vi "createCommandList.vi"(8 "error in (no error)":errorcluster, 10 "Parameters":u32[](array[numeric]), 11 "Burst in":refnum<class "Burst.lvclass">) -> (0 "error out":errorcluster, 2 "Commandlist":string, 3 "Burst out":refnum<class "Burst.lvclass">)   [LabVIEW 2013, in "Burst.lvclass"]
uses:
  Burst.lvclass
  TestInterface/TestInterface.lvclass
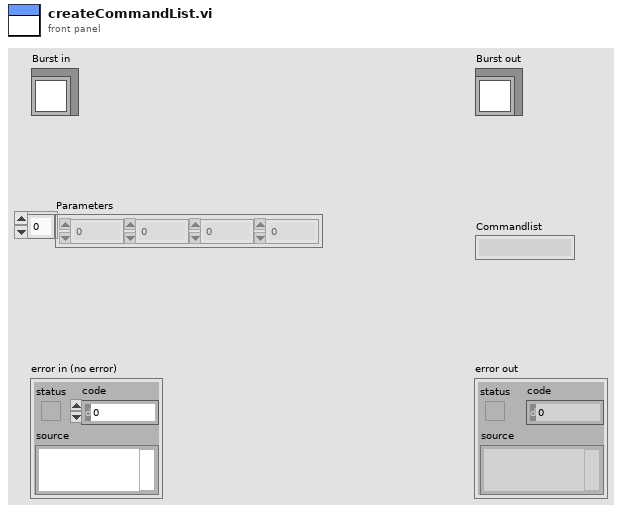
[diagram p1: front panel]
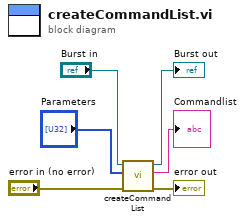
[diagram p0: block diagram]
diagram:
  n1 = call-parent "createCommandList.vi"("error in (no error)"="error in (no error)", "Parameters"="Parameters", "TestInterface in"="Burst in") -> ("error out"=→"error out":errorcluster, "Commandlist"=→"Commandlist":string, "TestInterface out"=→"Burst out":refnum<class "Burst.lvclass">)  [unwired: 6 in]
